vi "StimGenCleanup.vi"(8 "error in":errorcluster, 11 "stimulus specifier":T1) -> (0 "error out":errorcluster, 3 "stimulus specifier":T1)   [LabVIEW 2014]
uses:
  <vilib>/Instr/_visa.llb/VISA Flush IO Buffer Mask.ctl
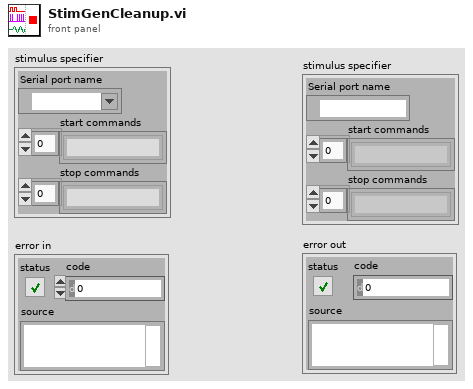
[diagram p1: front panel]
types:
  T1 = cluster{"Serial port name":refnum<visa-resource-name>, "start commands":string[], "stop commands":string[]}
  T2 = typedef "VISA Flush IO Buffer Mask.ctl" = u16
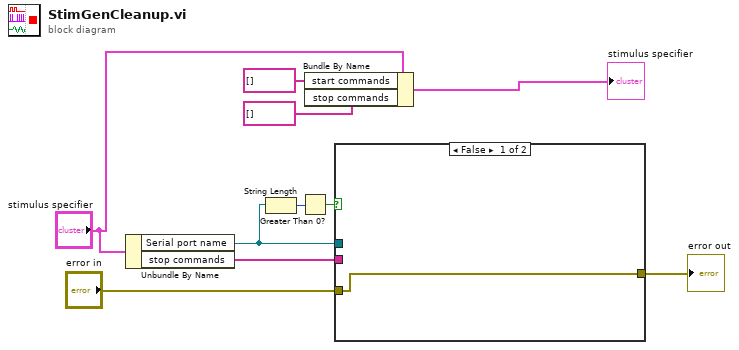
[diagram p0: block diagram]
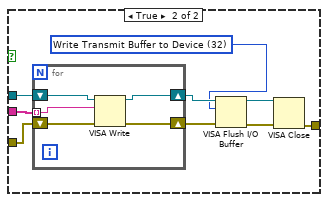
[diagram p2: hidden frame]
diagram:
  n1 = Unbundle By Name("stimulus specifier") -> ("Serial port name"=w1:refnum<visa-resource-name>, "stop commands"=w10:string[])
  n2 = String Length(string=w1) -> (length=w2:i32)
  n3 = Greater Than 0?(x=w2) -> (x > 0?=w3:bool)
  n4 = Bundle By Name(cluster="stimulus specifier", "start commands"=string[] [], "stop commands"=string[] []) -> (→"stimulus specifier":T1)
  n5 = case shown="False" w3 {
    tunnel: w10 -> [_ w20]
    tunnel: w1 -> [_ w19]
    tunnel: "error in" -> [w11 w18]
    tunnel: [w11 w13] -> w8
    frame False {
    }
    frame True {
      w12 = T2 32 items=["Flush Receive Buffer"=16, "Write Transmit Buffer to Device"=32, "Flush Receive Buffer (No I/O)"=64, "Flush Transmit Buffer"=128] ("Mask")
      n6 = for {
        tunnel: w20 -> [w24] mode=indexing
        shift-right: [w22] -> w17
        shift-left: w18 -> [w23]
        shift-right: [w21] -> w16
        shift-left: w19 -> [w25]
        n7 = VISA Write(VISA resource name=w25, write buffer=w24, error in (no error)=w23) -> (VISA resource name out=w21:refnum<visa-resource-name>, error out=w22:errorcluster)  [unwired: 1 out]
      }
      n8 = VISA Flush I/O Buffer(VISA resource name=w16, mask (16)=w12, error in (no error)=w17) -> (VISA resource name out=w15:refnum<visa-resource-name>, error out=w14:errorcluster)
      n9 = VISA Close(VISA resource name=w15, error in (no error)=w14) -> (error out=w13:errorcluster)
    }
  }
  "error out" <- w8
